vi "Magnet_Enable.vi"(8 "error in (no error)":errorcluster, 10 "Enable? (T)":bool=TRUE, 11 "VISA resource name":refnum<visa-resource-name>) -> (0 "error out":errorcluster, 3 "VISA resource name out":refnum<visa-resource-name>)   [LabVIEW 2010]
uses:
  <instrlib>/Keithley 24XX/Keithley 24XX.lvlib
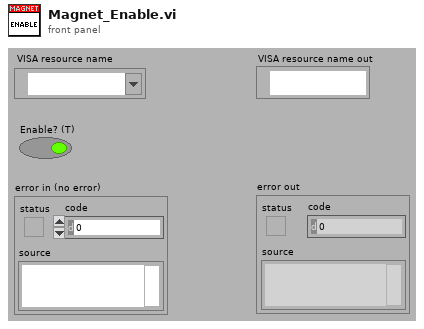
[diagram p1: front panel]
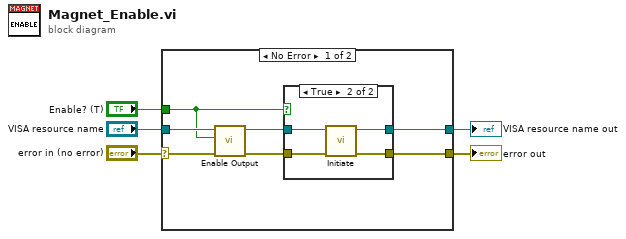
[diagram p0: block diagram]
diagram:
  n1 = case shown="No Error" "error in (no error)" {
    selector: "error in (no error)" -> [w9 w19]
    tunnel: "VISA resource name" -> [w10 w20]
    tunnel: "Enable? (T)" -> [w8 _]
    tunnel: [w7 w19] -> w2
    tunnel: [w6 w20] -> w1
    frame No Error {
      n2 = call <instrlib>:"Enable Output.vi"("error in (no error)"=w9, "Enable Output (T: Enable)"=w8, "VISA resource name"=w10) -> ("error out"=w11:errorcluster, "VISA resource name out"=w12:refnum<visa-resource-name>)  [unwired: 7 in]
      n3 = case shown="True" w8 {
        tunnel: w11 -> [w13 w18]
        tunnel: w12 -> [w14 w17]
        tunnel: [w13 w16] -> w7
        tunnel: [w14 w15] -> w6
        frame False {
        }
        frame True {
          n4 = call <instrlib>:"Initiate.vi"("error in (no error)"=w18, "VISA resource name"=w17) -> ("error out"=w16:errorcluster, "VISA resource name out"=w15:refnum<visa-resource-name>)  [unwired: 8 in]
        }
      }
    }
    frame Error {
    }
  }
  "error out" <- w2
  "VISA resource name out" <- w1
